vi "Lock Solenoid.vi"(10 "Value":T1, 11 "Enum":enum16{"Start", "Run", "End"}(ring)=enum."Run") -> ()   [LabVIEW 2012]
uses:
  TypeDefs/Solenoid Module 1.ctl
  <vilib>/Rock Robotics/WPI/Solenoid/WPI_SolenoidChannel.ctl
  <vilib>/Rock Robotics/SystemInterfaces/Typedef/FPGA_TypedefSolenoidModule.ctl
  <vilib>/Rock Robotics/WPI/Solenoid/WPI_SolenoidValue.ctl
  <vilib>/Rock Robotics/WPI/Solenoid/WPI_SolenoidOpenSingle.vi
  <vilib>/Rock Robotics/WPI/Solenoid/WPI_SolenoidSetEnum.vi
panel:
  in  "Solenoid Module 1":T2={"Lock Arm"=enum."Solenoid 1", "Shoot FWD"=enum."Solenoid 2", "Shoot REV"=enum."Solenoid 3", "Tip FWD"=enum."Solenoid 4", "Tip REV"=enum."Solenoid 5", "Unassigned"=enum."Solenoid 6", "Unassigned"=enum."Solenoid 7", "Unassigned"=enum."Solenoid 8", "Module"=enum."Solenoid Module 1"}
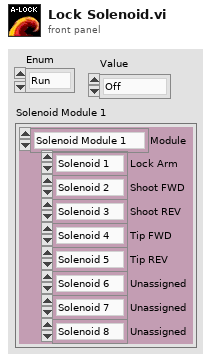
[diagram p1: front panel]
types:
  T1 = typedef "WPI_SolenoidValue.ctl" = enum16{"Off", "On", "Forward", "Reverse"}
  T2 = typedef "Solenoid Module 1.ctl" = cluster{"Lock Arm":T3, "Shoot FWD":T3, "Shoot REV":T3, "Tip FWD":T3, "Tip REV":T3, "Unassigned":T3, "Unassigned":T3, "Unassigned":T3, "Module":T4}
  T3 = typedef "WPI_SolenoidChannel.ctl" = enum8{"Solenoid 1", "Solenoid 2", "Solenoid 3", "Solenoid 4", "Solenoid 5", "Solenoid 6", "Solenoid 7", "Solenoid 8", "Invalid"}
  T4 = typedef "FPGA_TypedefSolenoidModule.ctl" = enum16{"Solenoid Module 1", "Solenoid Module 2"}
  T5 = typedef "WPI_SolenoidDevRef.ctl" = cluster{"DevStatus":errorcluster, "Solenoid Module":T4, "Forward Solenoid Channel":T3, "Reverse Solenoid Channel":T3}
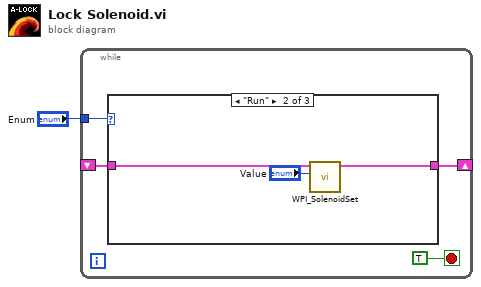
[diagram p0: block diagram]
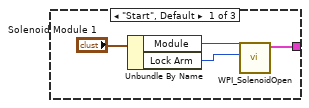
[diagram p2: hidden frame]
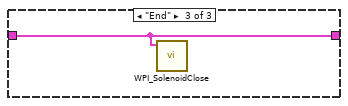
[diagram p3: hidden frame]
diagram:
  n1 = while {
    shift-right: [w5] -> _
    shift-left: _ -> [w3]
    tunnel: "Enum" -> [w4]
    stop <- TRUE stop-if-true
    n2 = case shown="\"Run\"" w4 {
      tunnel: [w9 w12 w13] -> w5
      tunnel: w3 -> [_ w11 w13]
      frame "Start", Default {
        n3 = Unbundle By Name("Solenoid Module 1") -> ("Module"=w8:T4, "Lock Arm"=w7:T3)
        n4 = call-poly <vilib>:"WPI_SolenoidOpen.vi"("Solenoid Channel"=w7, "Solenoid Module (Module 1)"=w8) -> ("SolenoidDevRef"=w9:T5)  [unwired: 8 in, 1 out]
      }
      frame "Run" {
        n5 = call-poly <vilib>:"WPI_SolenoidSet.vi"("Value"="Value", "SolenoidDevRef"=w11) -> ("SolenoidDevRef"=w12:T5)  [unwired: 8 in, 1 out]
      }
      frame "End" {
        n6 = call <vilib>:"WPI_SolenoidClose.vi"("SolenoidDevRef"=w13) -> ()  [unwired: 10 in, 1 out]
      }
    }
  }
